vi "GExplorer_Queue_GEA2_Multi.vi"(0 "Output String":string, 2 "State":T1(ring), 11 "error in (no error)":errorcluster) -> (15 "error out":errorcluster)   [LabVIEW 2016]
uses:
  typedefs/GExplorer_Data_Cluster_Multi.ctl
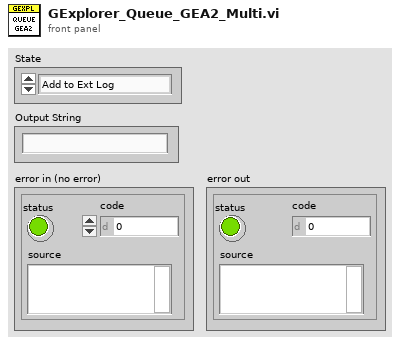
[diagram p1: front panel]
types:
  T1 = enum16{"Add to Ext Log", "Add to Int Log", "Clear", "Shutdown"}
  T2 = typedef "GExplorer_Data_Cluster_Multi.ctl" = cluster{"Data":variant, "State":enum16{"Add to Ext Log", "Add to Int Log", "Clear", "Shutdown"}}
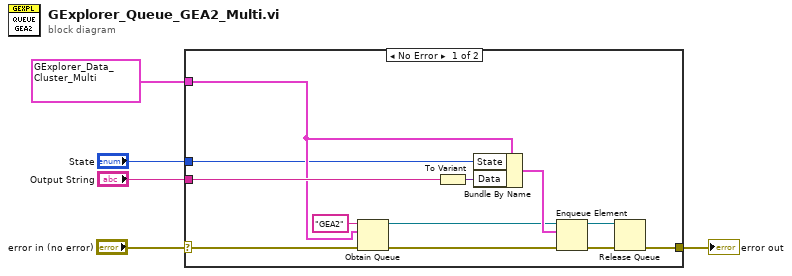
[diagram p0: block diagram]
diagram:
  n1 = case shown="No Error" "error in (no error)" {
    selector: "error in (no error)" -> [w14 w18]
    tunnel: [w8 w18] -> w5
    tunnel: "Output String" -> [w15 _]
    tunnel: T2 {"Data"=variant, "State"=enum."Add to Ext Log"} ("Data") -> [w7 _]
    tunnel: "State" -> [w6 _]
    frame No Error {
      n2 = Obtain Queue(name (unnamed)="GEA2", element data type=w7, error in (no error)=w14) -> (queue out=w12:refnum<queue>, error out=w13:errorcluster)  [unwired: 2 in, 1 out]
      n3 = To Variant(anything=w15) -> (Variant=w16:variant)
      n4 = Bundle By Name(cluster=w7, "State"=w6, "Data"=w16) -> (w17:T2)
      n5 = Enqueue Element(queue=w12, element=w17, error in (no error)=w13) -> (queue out=w9:refnum<queue>, error out=w10:errorcluster)  [unwired: 1 in, 1 out]
      n6 = Release Queue(queue=w9, error in (no error)=w10) -> (error out=w8:errorcluster)  [unwired: 1 in, 2 out]
    }
    frame Error {
    }
  }
  "error out" <- w5
